vi "FRCts20_Backend_FGVMessageReturnQueue.vi"(5 "Engine_Refnums":T2, 6 "Priority Message (F)":bool, 7 "Operation":T5, 8 "error in (no error)":errorcluster, 9 "Key":string, 10 "Message Value":string, 11 "Message Name":string) -> (0 "error out":errorcluster, 1 "Key (Duplicate)":string)   [LabVIEW 2014, in "FRCts20_Backend_Engine.lvlib"]
doc: "Enqueues requests to be handled by the AMC engine. The FGV stores the AMC message queues."
uses:
  FRCts20_Backend_Engine.lvlib
  FRCts20_Backend_FGVOperation.ctl
  FRCts20_Backend_EngineRefnums.ctl
  INI_Accessor/FRCts20_Backend_INI Controller.lvclass
  Dependencies/AMC/_SubVIs/TypeDefs/Message Queue.ctl
  Dependencies/AMC/_SubVIs/TypeDefs/Message.ctl
  Dependencies/Keyed Array/KeyedArray.ctl
  <vilib>/addons/database/Connection.llb/Conn ObjectReference.ctl
  Dependencies/AMC/AMC.lvlib
  Dependencies/Keyed Array/Tools_KeyedArray.lvlib
  <vilib>/addons/database/NI_Database_API.lvlib
panel:
  in  "Message Attributes":T1
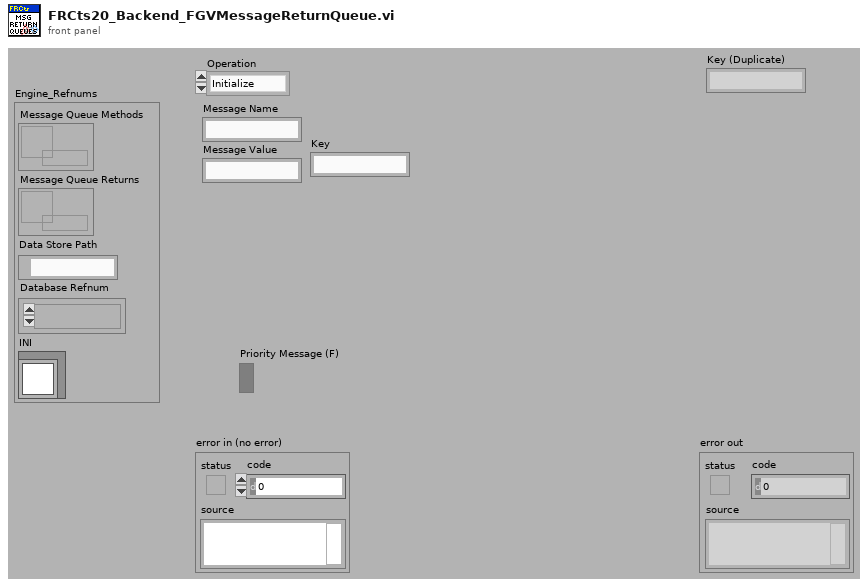
[diagram p1: front panel]
types:
  T1 = typedef "Tools_KeyedArray.lvlib/KeyedArray.ctl" = cluster{"keys":string[], "values":string[]}
  T2 = typedef "FRCts20_Backend_Engine.lvlib/FRCts20_Backend_EngineRefnums.ctl" = cluster{"Message Queue Methods":T3, "Message Queue Returns":T3, "Data Store Path":path, "Database Refnum":T4, "INI":refnum<class "FRCts20_Backend_INI Controller.lvclass">}
  T3 = typedef "AMC.lvlib/Message Queue.ctl" = refnum<queue>
  T4 = typedef "NI_Database_API.lvlib/Conn ObjectReference.ctl" = refnum<k1>
  T5 = typedef "FRCts20_Backend_Engine.lvlib/FRCts20_Backend_FGVOperation.ctl" = enum16{"Initialize", "EnqueueMessage", "EnqueueDataReturn", "FlushMessage", "FlushDataReturn"}
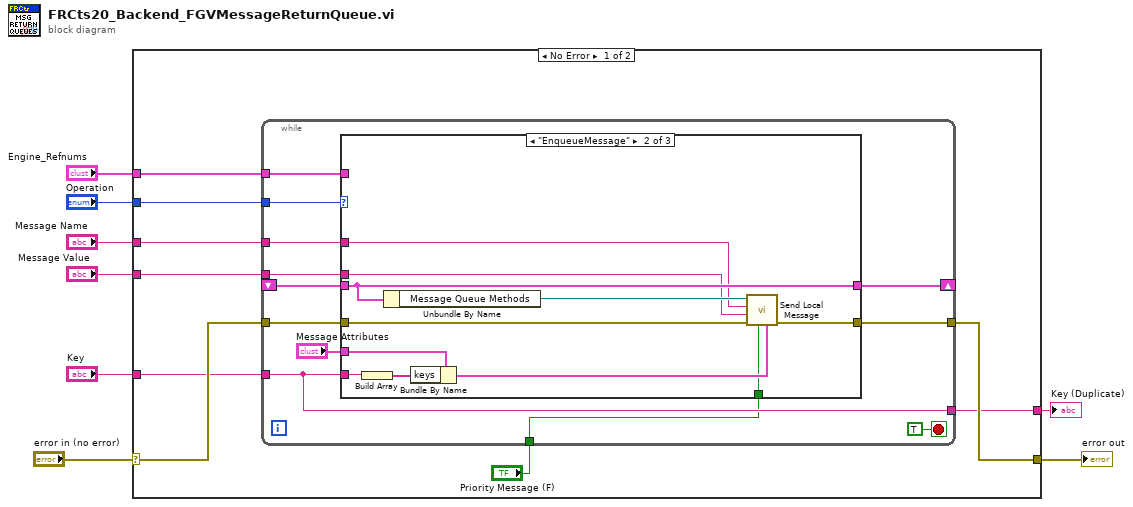
[diagram p0: block diagram]
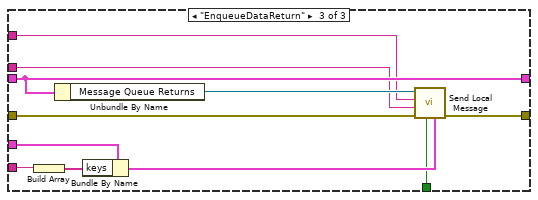
[diagram p3: hidden frame]
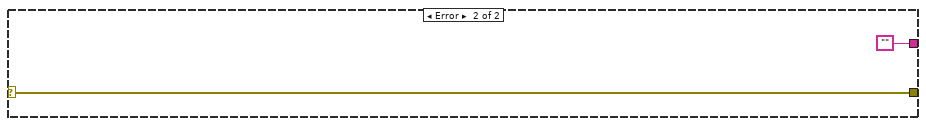
[diagram p4: hidden frame]
diagram:
  n1 = case shown="No Error" "error in (no error)" {
    selector: "error in (no error)" -> [w14 w55]
    tunnel: [w17 w55] -> w7
    tunnel: "Operation" -> [w16 _]
    tunnel: "Engine_Refnums" -> [w15 _]
    tunnel: "Key" -> [w13 _]
    tunnel: "Message Name" -> [w12 _]
    tunnel: "Message Value" -> [w11 _]
    tunnel: [w10 ""] -> w1
    frame No Error {
      n2 = while {
        tunnel: [w28] -> w17
        tunnel: w16 -> [w27]
        tunnel: w15 -> [w26]
        shift-right: [w25] -> _
        shift-left: _ -> [w24]
        tunnel: w14 -> [w23]
        tunnel: w13 -> [w19]
        tunnel: w12 -> [w22]
        tunnel: w11 -> [w21]
        tunnel: [w19] -> w10
        tunnel: "Priority Message (F)" -> [w18]
        stop <- TRUE stop-if-true
        n3 = case shown="\"EnqueueMessage\"" w27 {
          tunnel: [w30 w42 w53] -> w28
          tunnel: w26 -> [w31 _ _]
          tunnel: [w31 w39 w50] -> w25
          tunnel: w24 -> [_ w39 w50]
          tunnel: w23 -> [w30 w40 w51]
          tunnel: w19 -> [_ w38 w49]
          tunnel: w22 -> [_ w34 w45]
          tunnel: w21 -> [_ w35 w46]
          tunnel: "Message Attributes" -> [_ w33 w44]
          tunnel: w18 -> [_ w32 w43]
          frame "Initialize", Default {
          }
          frame "EnqueueMessage" {
            n4 = Build Array(w38) -> (w37:string[])
            n5 = Unbundle By Name(w39) -> ("Message Queue Methods"=w41:T3)
            n6 = Bundle By Name(cluster=w33, "keys"=w37) -> (w36:T1)
            n7 = call "Send Local Message.vi"("Message Attributes"=w36, "Priority Message (F)"=w32, "error in (no error)"=w40, "Message Value"=w35, "Message Name"=w34, "Message Queue in"=w41) -> ("error out"=w42:errorcluster)  [unwired: 4 in, 1 out]
          }
          frame "EnqueueDataReturn" {
            n8 = Build Array(w49) -> (w48:string[])
            n9 = Unbundle By Name(w50) -> ("Message Queue Returns"=w52:T3)
            n10 = Bundle By Name(cluster=w44, "keys"=w48) -> (w47:T1)
            n11 = call "Send Local Message.vi"("Message Attributes"=w47, "Priority Message (F)"=w43, "error in (no error)"=w51, "Message Value"=w46, "Message Name"=w45, "Message Queue in"=w52) -> ("error out"=w53:errorcluster)  [unwired: 4 in, 1 out]
          }
        }
      }
    }
    frame Error {
    }
  }
  "error out" <- w7
  "Key (Duplicate)" <- w1
